vi "Diagnostics.Channel.Engine.vi"(8 "error in":errorcluster, 11 "State Variables":T1={"Comm"=refnum, "Parameters"={"Name"="", "CAN"={"Interface"="", "Baud Rate"=0, "Diagnostic Protocol"=enum."GMLAN", "Transport Protocol"=enum."ISO TP - Normal Mode", "Transmit ID"=0, "Receive ID"=2, "Transmit Extension"=1, "Receive Extension"=255, "Receive UUDT ID"=0, "Enable Stream"=TRUE, "VW TP Channel ID"=1, "Fill Frame"=FALSE, "Fill Byte"=0, "Termination"=FALSE, "LIN Cluster"="", "NAD"=8, "IO Mode"=0, "Max DLC"=0, "FD Baud Rate"=2, "Timeout"=1, "FD ISO Mode"=0, "DoIP Address"="", "DoIP Source Address"=3584, "DoIP Dynamic Port"=TRUE, "DoIP Version"=2}, "986x"={"Enable"=FALSE, "RIO Device"="", "Bitfile"=path ""}, "Reads"=[], "Frames Lookup"=variant(enum16{"GMLAN", "KWP-2000", "UDS"} enum."GMLAN"), "Writes"=[], "DPIDs"=[], "DPID Lookup"=variant(u32 0), "DTC"={"Descriptor"={"DTC Byte Length"=1, "Status Byte Length"=1, "Add Data Byte Length"=1, "Byte Order"=enum."Motorola"}, "Value.Code"=[], "Value.String"=[], "Value.J2012String"=[], "Status.Code"=[], "Status.String"=[]}, "Created DTCs"=0, "Polls"=[], "Service Channels Status Lookup"=variant, "Trigger Lookup"=variant, "Security"={"Type"=enum."None", "Source DLL Path"=path "", "Target DLL Path"=path "", "Security Level"=0, "Static Master Key"="", "Max Key Length"=1, "Host IP Address"=""}, "Initial Comm State"=FALSE}, "ADCS Connection"={"Diag CAN Handle"=0, "Transport Protocol"=enum."ISO TP - Normal Mode", "Receive Address Extension"=0, "Transmit Address Extension"=0, "Receive CAN Id"=0, "Transmit CAN Id"=0, "Log Frames ?"=FALSE, "My TP Address"=0, "Other TP Address"=0, "T1"=0, "T2"=0, "T3"=0, "T4"=0, "Tx SN"=0, "Block Size"=0, "Rx SN"=0, "VW TP Initialized?"=FALSE, "Tx block no"=0, "baud rate"=0, "Interface"="", "Channel Diag CAN Handle"=0, "UDP Connection ID"=refnum, "TCP Connection ID"=refnum, "Target IP Addr"=0, "Source Address"=0, "Target Address"=0, "Send Header NACK?"=FALSE, "DLL Handle"=0, "NAD"=0, "Time Stamp read first"=0.0, "Time Stamp read last"=0.0, "Time Stamp write first"=0.0, "Time Stamp write last"=0.0, "Time Stamp write"=0.0, "Time Stamp read"=0.0, " I/O Mode"=0, "FD Baudrate"=0, "TX_DL"=8, "RX_DL"=8, "DoIP Protocol Version"=1, " Selected I/O Mode"=0, "TesterPresent Counter"=0, "TesterPresent Limit"=0, "TesterPresent Tick[ms]"=10, "TesterPresent RequireResponse?"=FALSE, "TesterPresent Stored Ref?"=FALSE, "TesterPresent Message"=[], "TesterPresent Task Handle"=0, "TesterPresent Semaphore"=refnum, "Response Plausibility Check"=1, "Default Version?"=TRUE, "Diagostic Globals"={"Timeout FC (Bs)"=250, "Timeout CF (Cr)"=250, "Timeout Diag Command"=1000, "Receive Block Size (BS)"=0, "Wait Time CF (STmin)"=5, "Max Waits (N_WFTmax)"=10, "Waits to Send (N_WAIT)"=0, "Time between Waits (TW)"=25, "Fill CAN Frames?"=TRUE, "Fill Byte"=255, "Invalid Response as Error?"=FALSE, "Max RspPending Count"=5, "VWTP Command Timeout"=50, "Transport Protocol"=enum."Diagnostics on IP", "Diag CAN Handle"=0, "DLL Handle"=0, "Timeout RspPending"=1000}, "Session-based Properties?"=FALSE}, "XNET References"={"Database"="", "GMLAN.DPID.Frame"="", "Cluster.Convert"=""}, "XNETEngine (GMLAN)"=refnum, "Process"=refnum, "Reads"=refnum, "Writes"=refnum, "Cmds"=refnum, "DTCs"=refnum, "DTC Count"=refnum, "Status"=refnum, "Triggers"=refnum, "CANConnected"=refnum, "LocalStop"=refnum, "LocalCommStatus"=refnum, "Service Channels Status"=refnum, "Settings"=refnum, "Streaming Refs"={"Addon"="", "Port"="", "Filter Ref"=refnum, "Default Filter"={"ID Filters"=[], "Direction Filter"=enum."Tx/Rx", "Type Filter"=enum."All"}, "Port Settings"={"Mode"=0, "Baud Rate"=0, "Termination"=0, "FD ISO Mode"=0, "FD Baud Rate"=0}}} {"Streaming Refs"."Port Settings"."FD ISO Mode" items=["ISO", "Non ISO", "ISO Legacy"]; "Streaming Refs"."Port Settings"."Termination" items=["Off", "On"]; "Streaming Refs"."Port Settings"."Mode" items=["CAN 2.0", "CAN FD", "CAN FD+BRS"]; "ADCS Connection"."Diagostic Globals"."Fill Byte" format="%x"; "ADCS Connection"."TesterPresent Message" format="%.0x"; "ADCS Connection"."Selected I/O Mode" items=["CAN", "CAN FD", "CAN FD+BRS", "ECU Determined"]; "ADCS Connection"."DoIP Protocol Version" items=["2010"=1, "2012"=2]; "ADCS Connection"."RX_DL" items=["8"=8, "12"=12, "16"=16, "20"=20, "24"=24, "32"=32, "48"=48, "64"=64]; "ADCS Connection"."TX_DL" items=["8"=8, "12"=12, "16"=16, "20"=20, "24"=24, "32"=32, "48"=48, "64"=64]; "ADCS Connection"."I/O Mode" items=["CAN", "CAN FD", "CAN FD+BRS", "Not yet determined"]; "Parameters"."Writes"."Signals"."Byte Order" items=["Little Endian", "Big Endian"]; "Parameters"."Writes"."Signals"."Data Type" items=["Signed", "Unsigned", "IEEE Float"]; "Parameters"."CAN"."DoIP Version" items=["2010"=1, "2012"=2]; "Parameters"."CAN"."DoIP Source Address" format="%.0x"; "Parameters"."CAN"."FD ISO Mode" items=["ISO", "Non ISO", "ISO Legacy"]; "Parameters"."CAN"."IO Mode" items=["CAN 2.0", "CAN FD", "CAN FD+BRS"]; "Parameters"."CAN"."Fill Byte" format="%.0x"; "Parameters"."CAN"."VW TP Channel ID" format="%.0x"; "Parameters"."CAN"."Receive UUDT ID" format="%.0x"; "Parameters"."CAN"."Receive Extension" format="%.0x"; "Parameters"."CAN"."Transmit Extension" format="%.0x"; "Parameters"."CAN"."Receive ID" format="%.0x"; "Parameters"."CAN"."Transmit ID" format="%.0x"; "Parameters"."Reads"."Signals"."Byte Order" items=["Little Endian", "Big Endian"]; "Parameters"."Reads"."Signals"."Data Type" items=["Signed", "Unsigned", "IEEE Float"]}) -> (0 "error out":errorcluster)   [LabVIEW 2019, in "Diagnostics Addon Engine.lvlib"]
uses:
  Diagnostics Addon Engine.lvlib
  Types/Diagnostics.State.ctl
  <vilib>/NI/NIVS Inline Async API/_VS Inline Async API/Process/Process.lvclass
  <vilib>/NI/NI VeriStand Addon Network Comm/Engine/VeriStand Comm.lvclass
  Addon Shared/Types/SysDef.Compile.ctl
  Addon Shared/Types/CAN.ctl
  Addon Shared/Types/CAN.Interface.ctl
  Addon Shared/Types/Protocol.ctl
  Addon Shared/Types/Transport.ctl
  Addon Shared/Types/986x.ctl
  Addon Shared/Types/Frame.Compile.ctl
  Addon Shared/Types/Type.ctl
  Addon Shared/Types/Signal.ctl
  Addon Shared/Types/DPID.ctl
  Addon Shared/Types/DPID.Rate.ctl
  Addon Shared/Types/DTC.Settings.ctl
  Addon Shared/Types/DTC.Descriptor.ctl
  Addon Shared/Types/Poll.Compiled.ctl
  Addon Shared/Types/Security.ctl
  Addon Shared/Types/Security.Type.ctl
  <vilib>/Automotive Diagnostic Command Set/Diagnostic Transport.llb/Diag Reference.ctl
  <vilib>/Automotive Diagnostic Command Set/Diagnostic Transport.llb/Transport Protocol Selector.ctl
  <vilib>/Automotive Diagnostic Command Set/Diagnostic Transport.llb/DoIP Protocol Version.ctl
  <vilib>/Automotive Diagnostic Command Set/Diagnostic Transport.llb/Diag Globals.ctl
  Types/XNET.Refs.ctl
  <vilib>/NI/AMC/Message Queue.ctl
  <vilib>/NI/AMC/Message.ctl
  <vilib>/NI/Tools/Keyed Array/KeyedArray.ctl
  <vilib>/NI/NIVS Inline Async API/_Data Access Engine/Data Access Engine/Types/Write.DVR.ctl
  <vilib>/NI/NIVS Inline Async API/_Data Access Engine/Access Type Classes/Write/Write.lvclass
  <vilib>/NI/NIVS Inline Async API/_Data Access Engine/Data Access Engine/Types/Read.DVR.ctl
  <vilib>/NI/NIVS Inline Async API/_Data Access Engine/Access Type Classes/Read/Read.lvclass
  <vilib>/NI/NIVS Inline Async API/_Data Access Engine/Data Access Engine/Types/ReadWrite.DVR.ctl
  <vilib>/NI/NIVS Inline Async API/_Data Access Engine/Access Type Classes/ReadWrite/ReadWrite.lvclass
  SubModules/CAN-Streaming-Support/Source/Addon/Addon Engine/Types/Engine Stream Refs.ctl
  SubModules/CAN-Streaming-Support/Source/Addon/Addon Shared/Types/Direction Filter.ctl
  SubModules/CAN-Streaming-Support/Source/Addon/Addon Shared/Types/Type Filter.ctl
  SubModules/CAN-Streaming-Support/Source/Addon/Addon Shared/Types/Filter Parameters.ctl
  SubModules/CAN-Streaming-Support/Source/Addon/Addon Engine/Types/Engine Stream Port Settings.ctl
  <vilib>/NI/NIVS Inline Async API/_Data Access Engine/Access Type Classes/ReadWrite/ReadWrite.lvclass/ReadWrite.ctl
  Addon Shared/Types/Trigger.Settings.ctl
  <vilib>/NI/NI VeriStand Addon Network Comm/Engine/VeriStand Comm.lvclass/VeriStand Comm.ctl
  <vilib>/NI/NIVS Inline Async API/_Data Access Engine/Access Type Classes/Read/Read.lvclass/Read.ctl
  Types/Diagnostics.Command.ctl
  Addon Shared/Types/Command.New.ctl
  <vilib>/NI/NIVS Inline Async API/_VS Inline Async API/Process/Process.lvclass/Process.ctl
  <vilib>/NI/NIVS Inline Async API/_Data Access Engine/Data Access Engine/Methods/ReadWrite.Data.Read.vi
  <vilib>/NI/NIVS Inline Async API/_Data Access Engine/Data Access Engine/Methods/ReadWrite.Data.Reset.vi
  <vilib>/NI/NIVS Inline Async API/_Data Access Engine/Data Access Engine/Methods/Read.Data.vi
  <vilib>/NI/NIVS Inline Async API/_Data Access Engine/Access Type Classes/ReadWrite/ReadWrite.ProcessData.Read.vi
  <vilib>/NI/NIVS Inline Async API/_Data Access Engine/Access Type Classes/ReadWrite/ReadWrite.ProcessData.Reset.vi
  <vilib>/NI/AMC/Send Local Message.vi
  Addon Shared/SubVIs/Format ECU Master Key to String.vi
  <vilib>/NI/AMC/Send Local Messages.vi
  <vilib>/NI/NIVS Inline Async API/_Data Access Engine/Access Type Classes/Read/Read.ProcessData.vi
  <vilib>/NI/NIVS Inline Async API/_VS Inline Async API/Error Handling Process/SubVIs/Error.ConvertArray.vi
  <vilib>/NI/AMC/Create Single Message.vi
  <vilib>/NI/AMC/Update Message Routing Info.vi
  <vilib>/NI/AMC/Create Multiple Messages.vi
  <vilib>/NI/AMC/Send Message.vi
  <vilib>/NI/NIVS Inline Async API/_Data Access Engine/Data Access Engine/Data Access Engine.lvclass
  Addon Shared/Diagnostics Addon Shared.lvlib
  <vilib>/NI/Tools/Keyed Array/Tools_KeyedArray.lvlib
  <vilib>/NI/AMC/AMC.lvlib
  <vilib>/addons/Automotive Diagnostic Command Set/NI_Automotive Diagnostic Command Set.lvlib
  SubModules/CAN-Streaming-Support/Source/Addon/Addon Engine/CAN Stream Support Engine.lvlib
  SubModules/CAN-Streaming-Support/Source/Addon/Addon Shared/CAN Stream Support Shared.lvlib
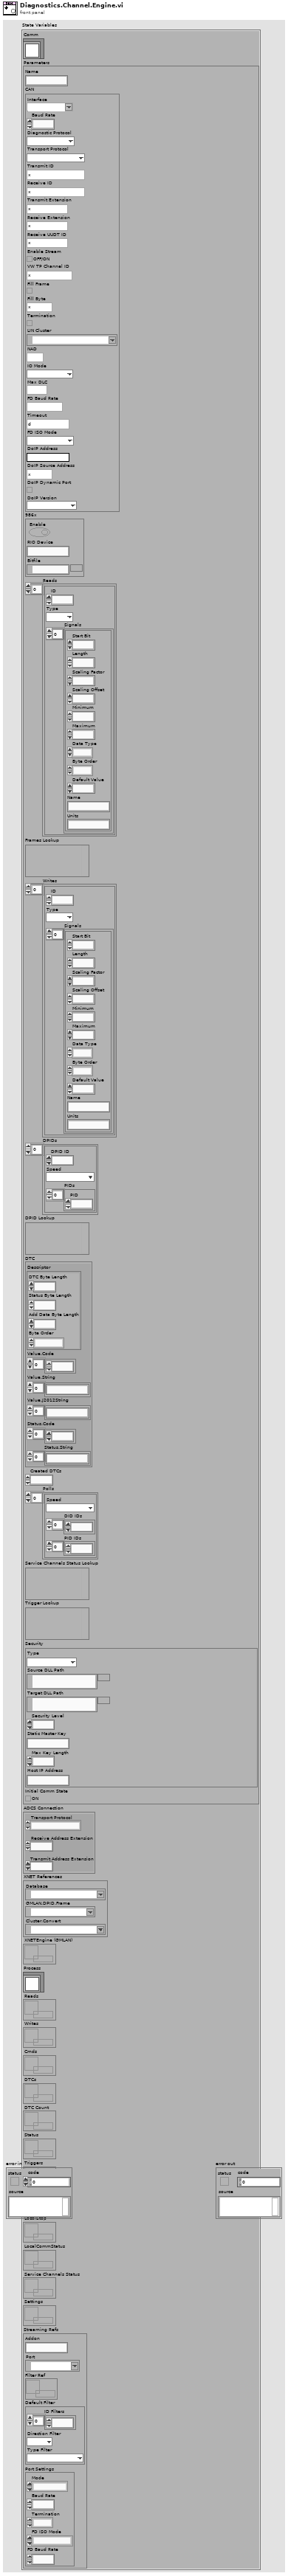
[diagram p1: front panel]
types:
  T1 = typedef "Diagnostics Addon Engine.lvlib/Diagnostics.State.ctl" = cluster{"Comm":refnum<class "VeriStand Comm.lvclass">, "Parameters":T2, "ADCS Connection":T18, "XNET References":T23, "XNETEngine (GMLAN)":T24, "Process":refnum<class "Process.lvclass">, "Reads":T25, "Writes":T26, "Cmds":T27, "DTCs":T25, "DTC Count":T25, "Status":T25, "Triggers":T27, "CANConnected":T25, "LocalStop":refnum<data-value>, "LocalCommStatus":refnum<data-value>, "Service Channels Status":T25, "Settings":T26, "Streaming Refs":T28}
  T2 = typedef "Diagnostics Addon Shared.lvlib/SysDef.Compile.ctl" = cluster{"Name":string, "CAN":T3, "986x":T7, "Reads":T8[], "Frames Lookup":variant, "Writes":T8[], "DPIDs":T11[], "DPID Lookup":variant, "DTC":T13, "Created DTCs":u32, "Polls":T15[], "Service Channels Status Lookup":variant, "Trigger Lookup":variant, "Security":T16, "Initial Comm State":bool}
  T3 = typedef "Diagnostics Addon Shared.lvlib/CAN.ctl" = cluster{"Interface":T4, "Baud Rate":u64, "Diagnostic Protocol":T5, "Transport Protocol":T6, "Transmit ID":u32, "Receive ID":u32, "Transmit Extension":u8, "Receive Extension":u8, "Receive UUDT ID":u32, "Enable Stream":bool, "VW TP Channel ID":u32, "Fill Frame":bool, "Fill Byte":u8, "Termination":bool, "LIN Cluster":refnum<k21>, "NAD":u8, "IO Mode":u32, "Max DLC":u16, "FD Baud Rate":u64, "Timeout":u32, "FD ISO Mode":u32, "DoIP Address":string, "DoIP Source Address":u16, "DoIP Dynamic Port":bool, "DoIP Version":u16}
  T4 = typedef "Diagnostics Addon Shared.lvlib/CAN.Interface.ctl" = string
  T5 = typedef "Diagnostics Addon Shared.lvlib/Protocol.ctl" = enum16{"GMLAN", "KWP-2000", "UDS", "User-Defined"}
  T6 = typedef "Diagnostics Addon Shared.lvlib/Transport.ctl" = enum16{"ISO TP - Normal Mode", "ISO TP - Mixed Mode", "VW TP 2.0", "Diagnostics on IP", "ISO TP LIN"}
  T7 = typedef "Diagnostics Addon Shared.lvlib/986x.ctl" = cluster{"Enable":bool, "RIO Device":string, "Bitfile":path}
  T8 = typedef "Diagnostics Addon Shared.lvlib/Frame.Compile.ctl" = cluster{"ID":u32, "Type":T9, "Signals":T10[]}
  T9 = typedef "Diagnostics Addon Shared.lvlib/Type.ctl" = enum16{"DID", "CDID", "PID", "CPID", "Read Memory", "Write Memory", "IO Control", "Routine Start", "Routine Request", "Routine Stop", "User Defined", "DTC Control", "Clear DTCs", "Read DTCs", "Start DTCs", "DTC Change Count", "Tester Present", "Unlock ECU", "Reset ECU", "Diag Session Control", "Communication Control", "DPID Control", "Poll Control", "Diag Comm Port Control"}
  T10 = typedef "Diagnostics Addon Shared.lvlib/Signal.ctl" = cluster{"Start Bit":u32, "Length":u32, "Scaling Factor":dbl, "Scaling Offset":dbl, "Minimum":dbl, "Maximum":dbl, "Data Type":u32, "Byte Order":u32, "Default Value":dbl, "Name":string, "Units":string}
  T11 = typedef "Diagnostics Addon Shared.lvlib/DPID.ctl" = cluster{"DPID ID":u8, "Speed":T12, "PIDs":u16[]}
  T12 = typedef "Diagnostics Addon Shared.lvlib/DPID.Rate.ctl" = enum16{"Slow", "Medium", "Fast"}
  T13 = typedef "Diagnostics Addon Shared.lvlib/DTC.Settings.ctl" = cluster{"Descriptor":T14, "Value.Code":dbl[], "Value.String":string[], "Value.J2012String":string[], "Status.Code":dbl[], "Status.String":string[]}
  T14 = typedef "Diagnostics Addon Shared.lvlib/DTC.Descriptor.ctl" = cluster{"DTC Byte Length":i32, "Status Byte Length":i32, "Add Data Byte Length":i32, "Byte Order":enum16{"Motorola", "Intel"}}
  T15 = typedef "Diagnostics Addon Shared.lvlib/Poll.Compiled.ctl" = cluster{"Speed":T12, "DID IDs":u32[], "PID IDs":u32[]}
  T16 = typedef "Diagnostics Addon Shared.lvlib/Security.ctl" = cluster{"Type":T17, "Source DLL Path":path, "Target DLL Path":path, "Security Level":u8, "Static Master Key":string, "Max Key Length":u32, "Host IP Address":string}
  T17 = typedef "Diagnostics Addon Shared.lvlib/Security.Type.ctl" = enum16{"None", "SeedKey DLL", "MasterKey (Channel)", "MasterKey (Static)", "SeedKey DLL (Windows)"}
  T18 = typedef "NI_Automotive Diagnostic Command Set.lvlib/Diag Reference.ctl" = cluster{"Diag CAN Handle":u32, "Transport Protocol":T19, "Receive Address Extension":u8, "Transmit Address Extension":u8, "Receive CAN Id":u32, "Transmit CAN Id":u32, "Log Frames ?":bool, "My TP Address":u8, "Other TP Address":u8, "T1":u16, "T2":u16, "T3":u16, "T4":u16, "Tx SN":u8, "Block Size":u8, "Rx SN":u8, "VW TP Initialized?":bool, "Tx block no":u8, "baud rate":u64, "Interface":string, "Channel Diag CAN Handle":u32, "UDP Connection ID":refnum<k16>, "TCP Connection ID":refnum<k5>, "Target IP Addr":u32, "Source Address":u16, "Target Address":u16, "Send Header NACK?":bool, "DLL Handle":u32, "NAD":u8, "Time Stamp read first":dbl, "Time Stamp read last":dbl, "Time Stamp write first":dbl, "Time Stamp write last":dbl, "Time Stamp write":dbl, "Time Stamp read":dbl, " I/O Mode":u32, "FD Baudrate":u64, "TX_DL":u16, "RX_DL":u16, "DoIP Protocol Version":T20, " Selected I/O Mode":u32, "TesterPresent Counter":u32, "TesterPresent Limit":u32, "TesterPresent Tick[ms]":i32, "TesterPresent RequireResponse?":bool, "TesterPresent Stored Ref?":bool, "TesterPresent Message":u8[], "TesterPresent Task Handle":i32, "TesterPresent Semaphore":T21, "Response Plausibility Check":u32, "Default Version?":bool, "Diagostic Globals":T22, "Session-based Properties?":bool}
  T19 = typedef "NI_Automotive Diagnostic Command Set.lvlib/Transport Protocol Selector.ctl" = enum16{"ISO TP - Normal Mode", "ISO TP - Mixed Mode", "VW TP 2.0", "Diagnostics on IP", "ISO TP LIN"}
  T20 = typedef "NI_Automotive Diagnostic Command Set.lvlib/DoIP Protocol Version.ctl" = u8
  T21 = typedef "Semaphore RefNum" = refnum<k1>
  T22 = typedef "NI_Automotive Diagnostic Command Set.lvlib/Diag Globals.ctl" = cluster{"Timeout FC (Bs)":u32, "Timeout CF (Cr)":u32, "Timeout Diag Command":u32, "Receive Block Size (BS)":u8, "Wait Time CF (STmin)":u8, "Max Waits (N_WFTmax)":u8, "Waits to Send (N_WAIT)":i32, "Time between Waits (TW)":u32, "Fill CAN Frames?":bool, "Fill Byte":u32, "Invalid Response as Error?":bool, "Max RspPending Count":u32, "VWTP Command Timeout":u32, "Transport Protocol":T19, "Diag CAN Handle":u32, "DLL Handle":u32, "Timeout RspPending":u32}
  T23 = typedef "Diagnostics Addon Engine.lvlib/XNET.Refs.ctl" = cluster{"Database":refnum<k21>, "GMLAN.DPID.Frame":refnum<k21>, "Cluster.Convert":refnum<k21>}
  T24 = typedef "AMC.lvlib/Message Queue.ctl" = refnum<queue>
  T25 = typedef "Data Access Engine.lvlib/Data Access Engine.lvclass/Write.DVR.ctl" = refnum<data-value>
  T26 = typedef "Data Access Engine.lvlib/Data Access Engine.lvclass/Read.DVR.ctl" = refnum<data-value>
  T27 = typedef "Data Access Engine.lvlib/Data Access Engine.lvclass/ReadWrite.DVR.ctl" = refnum<data-value>
  T28 = typedef "CAN Stream Support Engine.lvlib/Engine Stream Refs.ctl" = cluster{"Addon":string, "Port":refnum<k21>, "Filter Ref":refnum<data-value>, "Default Filter":T29, "Port Settings":T32}
  T29 = typedef "CAN Stream Support Shared.lvlib/Filter Parameters.ctl" = cluster{"ID Filters":u32[], "Direction Filter":T30, "Type Filter":T31}
  T30 = typedef "CAN Stream Support Shared.lvlib/Direction Filter.ctl" = enum16{"Tx/Rx", "Rx", "Tx"}
  T31 = typedef "CAN Stream Support Shared.lvlib/Type Filter.ctl" = enum16{"All", "CAN Data", "CAN Remote", "CAN Bus Error", "CAN 2.0 Data", "CAN FD Data", "CAN FD+BRS Data", "J1939 Data", "Delay", "Log Trigger", "Start Trigger"}
  T32 = typedef "CAN Stream Support Engine.lvlib/Engine Stream Port Settings.ctl" = cluster{"Mode":u32, "Baud Rate":u64, "Termination":u32, "FD ISO Mode":u32, "FD Baud Rate":u64}
  T33 = typedef "Diagnostics Addon Shared.lvlib/Trigger.Settings.ctl" = cluster{"Type":T9, "ID":u32, "Settings?":bool, "Index":i32, "Length":i32}
  T34 = typedef "Diagnostics Addon Engine.lvlib/Diagnostics.Command.ctl" = enum8{"None", "Clear Status Channels", "Read DIDs", "Read DID", "Write DID", "Read PIDs", "Read PID", "Write CPID", "Write Memory", "Read Memory", "Input Output Control", "Start Routine", "Request Routine Status", "Stop Routine", "Configure and Start DPIDs", "Stop DPIDs", "Start DTCs", "Read DTCs", "Clear DTCs", "Control DTC", "Read Failure Record Parameters", "Enable Change DTC Count", "Disable Change DTC Count", "Restart Communication", "Close Communication", "Force Tester Present", "Enable Repeating Tester Present", "Disable Repeating Tester Present", "Unlock ECU", "ECU Reset", "Enable Diagnostic Session", "Disable Diagnostic Session", "Disable Normal Communication", "Return To Normal Mode", "Pass Thru Channel Based", "Start Polling", "Stop Polling"}
  T35 = typedef "Diagnostics Addon Shared.lvlib/Command.New.ctl" = enum8{"None", "Clear Status Channels", "Read All DIDs", "Read All PIDs", "Configure and Start DPIDs", "Stop DPIDs"}
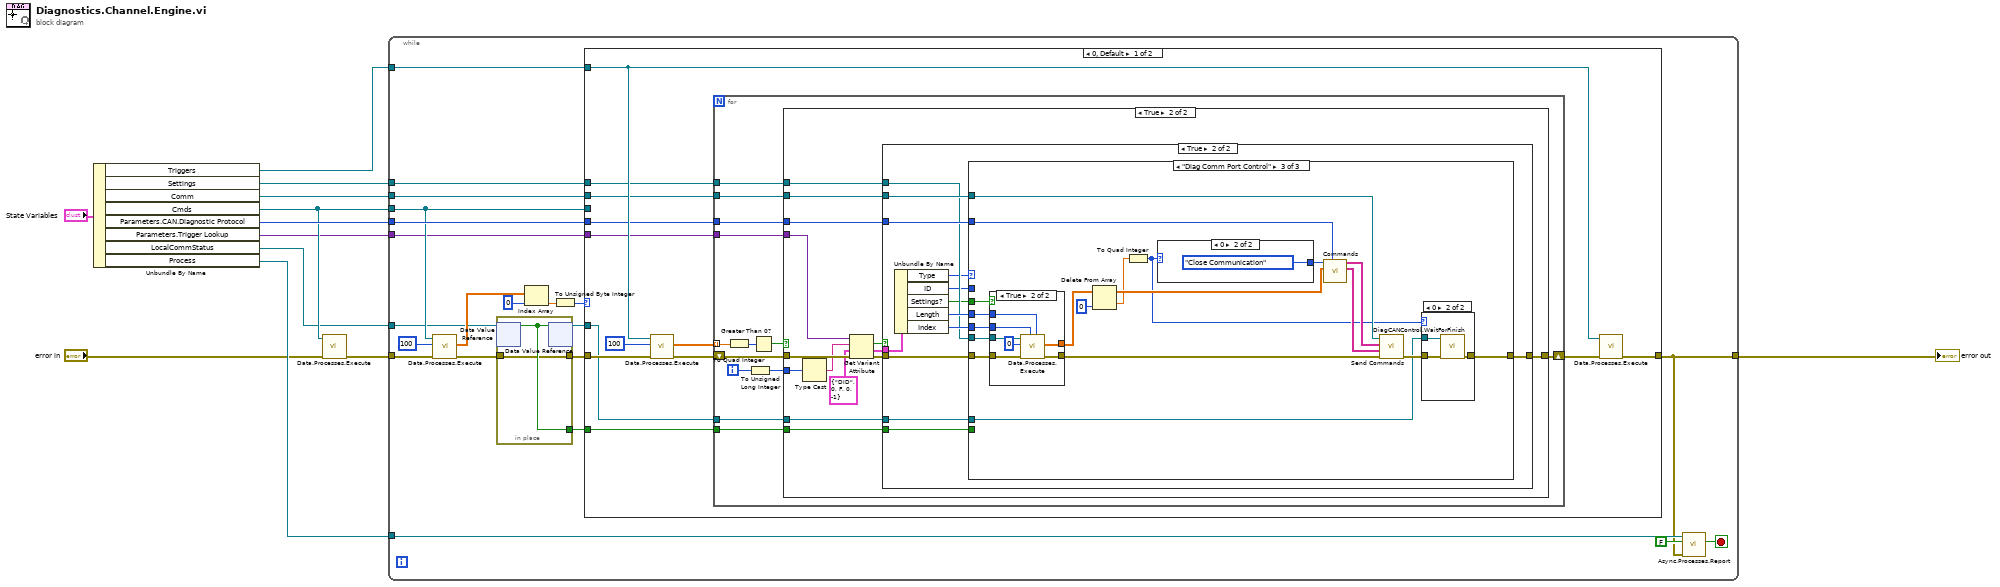
[diagram p0: block diagram]
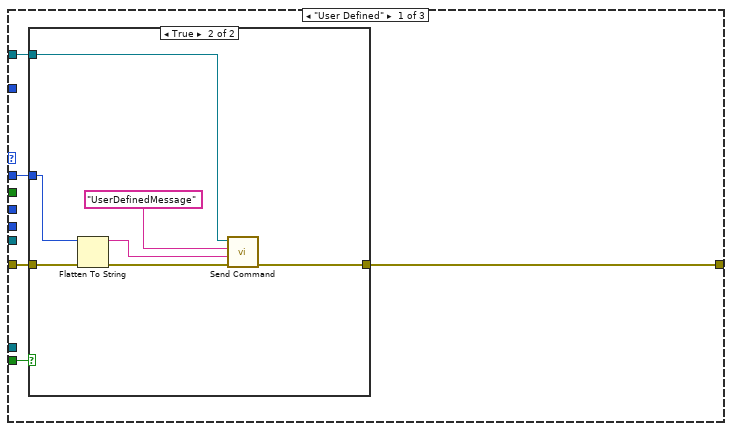
[diagram p4: hidden frame]
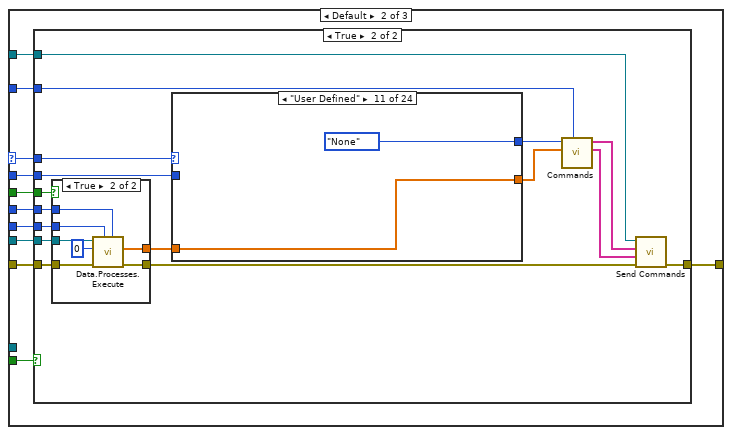
[diagram p6: hidden frame]
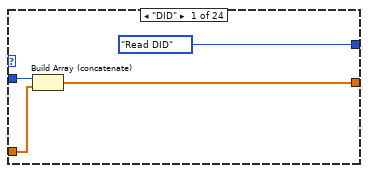
[diagram p8: hidden frame]
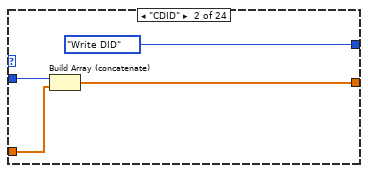
[diagram p9: hidden frame]
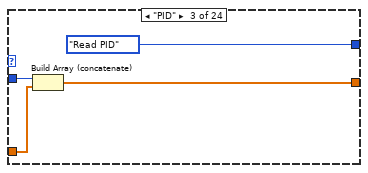
[diagram p10: hidden frame]
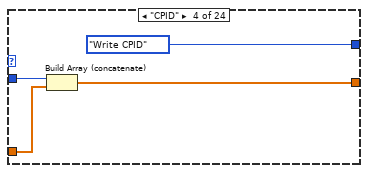
[diagram p11: hidden frame]
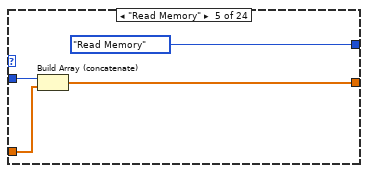
[diagram p12: hidden frame]
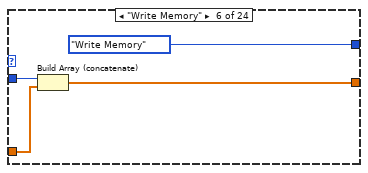
[diagram p13: hidden frame]
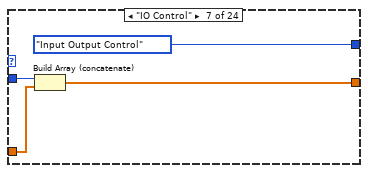
[diagram p14: hidden frame]
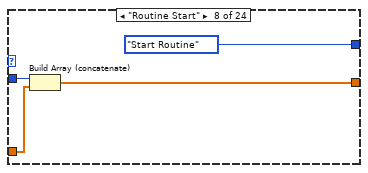
[diagram p15: hidden frame]
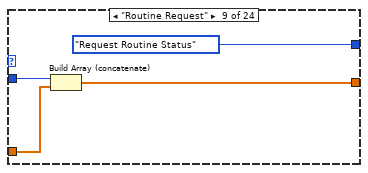
[diagram p16: hidden frame]
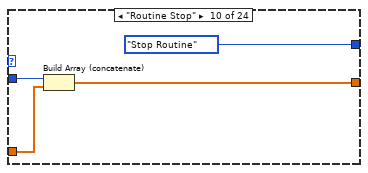
[diagram p17: hidden frame]
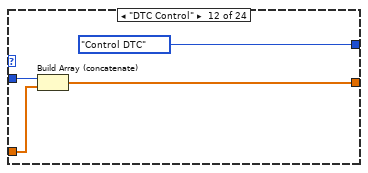
[diagram p18: hidden frame]
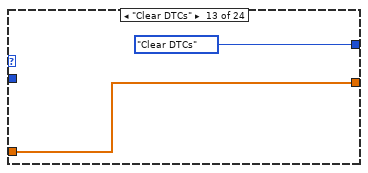
[diagram p19: hidden frame]
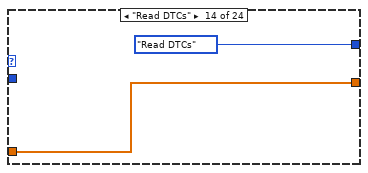
[diagram p20: hidden frame]
diagram:
  n1 = Unbundle By Name("State Variables") -> ("Triggers"=w7:T27, "Settings"=w2:T26, "Comm"=w9:refnum<class "VeriStand Comm.lvclass">, "Cmds"=w4:T27, "Parameters.CAN.Diagnostic Protocol"=w8:T5, "Parameters.Trigger Lookup"=w1:variant, "LocalCommStatus"=w3:refnum<data-value>, "Process"=w11:refnum<class "Process.lvclass">)
  n2 = call-poly <vilib>:"Data.Processes.Execute.vi"("error in (no error)"="error in", "Ref"=w4) -> ("error out"=w5:errorcluster)  [unwired: 8 in, 1 out]
  n3 = while {
    tunnel: w4 -> [w25]
    tunnel: w11 -> [w30]
    tunnel: [w24] -> w10
    tunnel: w5 -> [w26]
    tunnel: w9 -> [w33]
    tunnel: w8 -> [w32]
    tunnel: w7 -> [w29]
    tunnel: w3 -> [w19]
    tunnel: w2 -> [w17]
    tunnel: w1 -> [w16]
    stop <- w23 stop-if-true
    n4 = call-poly <vilib>:"Data.Processes.Execute.vi"("error in (no error)"=w26, "timeout ms"=100 ("timeout in ms (0)"), "Ref"=w25) -> ("error out"=w21:errorcluster, "Data"=w27:dbl[])  [unwired: 5 in, 2 out]
    n5 = in-place {
      in-place-border: [w35] -> w20
      in-place-border: [w34] -> w22
      in-place-border: w21 -> [w34]
      n6 = in-place-dvr #1(w19) -> (w35:bool)  [unwired: 1 out]
      n7 = in-place-dvr #1(w35) -> (w18:refnum<data-value>)  [unwired: 1 out]
    }
    n8 = Index Array(array=w27, index=0) -> (element=w14:dbl)
    n9 = To Unsigned Byte Integer(number=w14) -> (unsigned 8bit integer=w13:u8)
    n10 = case shown="0, Default" w13 {
      selector: w13 -> [_ w294]
      tunnel: w22 -> [w43 w297]
      tunnel: [w41 w292] -> w24
      tunnel: w33 -> [w42 w296]
      tunnel: w32 -> [w40 w295]
      tunnel: w29 -> [w44 _]
      tunnel: w25 -> [_ w289]
      tunnel: w20 -> [w36 w291]
      tunnel: w18 -> [w37 _]
      tunnel: w17 -> [w39 _]
      tunnel: w16 -> [w38 _]
      frame 0, Default {
        n11 = call-poly <vilib>:"Data.Processes.Execute.vi"("error in (no error)"=w43, "timeout ms"=100 ("timeout in ms (0)"), "Ref"=w44) -> ("error out"=w47:errorcluster, "Data"=w46:dbl[])  [unwired: 5 in, 2 out]
        n12 = for {
          shift-right: [w57] -> w45
          shift-left: w47 -> [w58]
          tunnel: w46 -> [w61] mode=indexing
          tunnel: w40 -> [w56]
          tunnel: w42 -> [w55]
          tunnel: w39 -> [w54]
          tunnel: w38 -> [w53]
          tunnel: w37 -> [w51]
          tunnel: w36 -> [w50]
          i -> [w52]
          n13 = To Quad Integer(1:w61) -> (0:w60:i64)
          n14 = To Unsigned Long Integer(number=w52) -> (unsigned 32bit integer=w49:u32)
          n15 = Greater Than 0?(x=w60) -> (x > 0?=w59:bool)
          n16 = case shown="True" w59 {
            tunnel: w58 -> [w62 w76]
            tunnel: [w62 w69] -> w57
            tunnel: w49 -> [_ w75]
            tunnel: w56 -> [_ w70]
            tunnel: w55 -> [_ w68]
            tunnel: w54 -> [_ w67]
            tunnel: w53 -> [_ w66]
            tunnel: w51 -> [_ w64]
            tunnel: w50 -> [_ w63]
            frame False {
            }
            frame True {
              n17 = Type Cast(x=w75) -> (*(type *) &x=w74:string)  [unwired: 1 in]
              n18 = Get Variant Attribute(Variant=w66, name=w74, default value (empty Variant)=T33 {"Type"=enum."DID", "ID"=0, "Settings?"=FALSE, "Index"=0, "Length"=-1}, error in=w76) -> (found=w65:bool, value=w72:T33, error out=w71:errorcluster)  [unwired: 1 out]
              n19 = case shown="True" w65 {
                tunnel: w72 -> [_ w90]
                tunnel: w71 -> [w77 w87]
                tunnel: w70 -> [_ w86]
                tunnel: [w77 w85] -> w69
                tunnel: w68 -> [_ w84]
                tunnel: w67 -> [_ w83]
                tunnel: w64 -> [_ w79]
                tunnel: w63 -> [_ w78]
                frame False {
                }
                frame True {
                  n20 = Unbundle By Name(w90) -> ("Type"=w81:T9, "ID"=w80:u32, "Settings?"=w82:bool, "Length"=w88:i32, "Index"=w89:i32)
                  n21 = case shown="\"Diag Comm Port Control\"" w81 {
                    selector: w81 -> [_ w106 _]
                    tunnel: w89 -> [_ w114 w274]
                    tunnel: w88 -> [_ w113 w273]
                    tunnel: w87 -> [w92 w112 w272]
                    tunnel: w86 -> [_ w111 w270]
                    tunnel: [w95 w110 w258] -> w85
                    tunnel: w84 -> [w94 w109 w267]
                    tunnel: w83 -> [_ w108 w266]
                    tunnel: w82 -> [_ w107 w265]
                    tunnel: w80 -> [w93 w105 _]
                    tunnel: w79 -> [_ _ w257]
                    tunnel: w78 -> [w91 w104 _]
                    frame "User Defined" {
                      n22 = case shown="True" w91 {
                        tunnel: [w96 w103] -> w95
                        tunnel: w94 -> [_ w102]
                        tunnel: w93 -> [_ w100]
                        tunnel: w92 -> [w96 w98]
                        frame False {
                        }
                        frame True {
                          n23 = Flatten To String(anything=w100, error in (no error)=w98) -> (data string=w97:string, error out=w99:errorcluster)  [unwired: 2 in, 1 out]
                          n24 = call <vilib>:"Send Command.vi"("error in (no error)"=w99, "message value"=w97, "message name"="UserDefinedMessage", "VeriStand Comm in"=w102) -> ("error out"=w103:errorcluster)  [unwired: 6 in, 1 out]
                        }
                      }
                    }
                    frame Default {
                      n25 = case shown="True" w104 {
                        tunnel: w114 -> [_ w131]
                        tunnel: w113 -> [_ w130]
                        tunnel: w112 -> [w115 w129]
                        tunnel: w111 -> [_ w127]
                        tunnel: [w115 w126] -> w110
                        tunnel: w109 -> [_ w123]
                        tunnel: w108 -> [_ w122]
                        tunnel: w107 -> [_ w121]
                        tunnel: w106 -> [_ w120]
                        tunnel: w105 -> [_ w117]
                        frame False {
                        }
                        frame True {
                          n26 = case shown="True" w121 {
                            tunnel: w131 -> [_ w255]
                            tunnel: w130 -> [_ w254]
                            tunnel: w129 -> [w248 w253]
                            tunnel: [_ w251] -> w118
                            tunnel: [w248 w250] -> w128
                            tunnel: w122 -> [_ w249]
                            frame False {
                            }
                            frame True {
                              n27 = call-poly <vilib>:"Data.Processes.Execute.vi"("length"=w254, "index"=w255, "error in (no error)"=w253, "timeout ms"=0, "Ref"=w249) -> ("error out"=w250:errorcluster, "Values"=w251:dbl[])  [unwired: 4 in, 1 out]
                            }
                          }
                          n28 = case shown="\"User Defined\"" w120 {
                            tunnel: [Diagnostics.Command."Read DID" ("Enum") Diagnostics.Command."Write DID" ("Enum") Diagnostics.Command."Read PID" ("Enum") Diagnostics.Command."Write CPID" ("Enum") Diagnostics.Command."Read Memory" ("Enum") Diagnostics.Command."Write Memory" ("Enum") Diagnostics.Command."Input Output Control" ("Enum") Diagnostics.Command."Start Routine" ("Enum") Diagnostics.Command."Request Routine Status" ("Enum") Diagnostics.Command."Stop Routine" ("Enum") Diagnostics.Command."None" ("Enum") Diagnostics.Command."Control DTC" ("Enum") Diagnostics.Command."Clear DTCs" ("Enum") Diagnostics.Command."Read DTCs" ("Enum") Diagnostics.Command."Start DTCs" ("Enum") w189 w192 Diagnostics.Command."Unlock ECU" ("Enum") Diagnostics.Command."ECU Reset" ("Enum") w204 w212 w223 w233 w240] -> w119
                            tunnel: w118 -> [w133 w137 w141 w145 w149 w153 w157 w161 w165 w169 w172 w175 w178 w180 w182 w188 w194 w200 w202 w206 w214 w224 w234 w242]
                            tunnel: w117 -> [w134 w138 w142 w146 w150 w154 w158 w162 w166 w170 _ w176 _ _ _ _ _ _ _ _ _ w222 w232 _]
                            tunnel: [w132 w136 w140 w144 w148 w152 w156 w160 w164 w168 w172 w174 w178 w180 w182 w186 w193 w200 w202 w205 w213 w220 w230 w241] -> w116
                            frame "DID" {
                              n29 = Build Array (concatenate)(w134, w133) -> (w132:dbl[])
                            }
                            frame "CDID" {
                              n30 = Build Array (concatenate)(w138, w137) -> (w136:dbl[])
                            }
                            frame "PID" {
                              n31 = Build Array (concatenate)(w142, w141) -> (w140:dbl[])
                            }
                            frame "CPID" {
                              n32 = Build Array (concatenate)(w146, w145) -> (w144:dbl[])
                            }
                            frame "Read Memory" {
                              n33 = Build Array (concatenate)(w150, w149) -> (w148:dbl[])
                            }
                            frame "Write Memory" {
                              n34 = Build Array (concatenate)(w154, w153) -> (w152:dbl[])
                            }
                            frame "IO Control" {
                              n35 = Build Array (concatenate)(w158, w157) -> (w156:dbl[])
                            }
                            frame "Routine Start" {
                              n36 = Build Array (concatenate)(w162, w161) -> (w160:dbl[])
                            }
                            frame "Routine Request" {
                              n37 = Build Array (concatenate)(w166, w165) -> (w164:dbl[])
                            }
                            frame "Routine Stop" {
                              n38 = Build Array (concatenate)(w170, w169) -> (w168:dbl[])
                            }
                            frame "User Defined" {
                            }
                            frame "DTC Control" {
                              n39 = Build Array (concatenate)(w176, w175) -> (w174:dbl[])
                            }
                            frame "Clear DTCs" {
                            }
                            frame "Read DTCs" {
                            }
                            frame "Start DTCs" {
                            }
                            frame "DTC Change Count" {
                              n40 = Delete From Array(array=w188, index=0) -> (deleted portion=w185:dbl, array with subset deleted=w186:dbl[])  [unwired: 1 in]
                              n41 = To Quad Integer(1:w185) -> (0:w184:i64)
                              n42 = case shown="0" w184 {
                                tunnel: [Diagnostics.Command."Enable Change DTC Count" ("Enum") Diagnostics.Command."Disable Change DTC Count" ("Enum")] -> w189
                                frame Default {
                                }
                                frame 0 {
                                }
                              }
                            }
                            frame "Tester Present" {
                              n43 = Delete From Array(array=w194, index=0) -> (deleted portion=w196:dbl, array with subset deleted=w193:dbl[])  [unwired: 1 in]
                              n44 = To Quad Integer(1:w196) -> (0:w195:i64)
                              n45 = case shown="0" w195 {
                                tunnel: [Diagnostics.Command."Enable Repeating Tester Present" ("Enum") Diagnostics.Command."Disable Repeating Tester Present" ("Enum")] -> w192
                                frame Default {
                                }
                                frame 0 {
                                }
                              }
                            }
                            frame "Unlock ECU" {
                            }
                            frame "Reset ECU" {
                            }
                            frame "Diag Session Control" {
                              n46 = Delete From Array(array=w206, index=0) -> (deleted portion=w208:dbl, array with subset deleted=w205:dbl[])  [unwired: 1 in]
                              n47 = To Quad Integer(1:w208) -> (0:w207:i64)
                              n48 = case shown="Default" w207 {
                                tunnel: [Diagnostics.Command."Enable Diagnostic Session" ("Enum") Diagnostics.Command."Disable Diagnostic Session" ("Enum")] -> w204
                                frame Default {
                                }
                                frame 0 {
                                }
                              }
                            }
                            frame "Communication Control" {
                              n49 = Delete From Array(array=w214, index=0) -> (deleted portion=w216:dbl, array with subset deleted=w213:dbl[])  [unwired: 1 in]
                              n50 = To Quad Integer(1:w216) -> (0:w215:i64)
                              n51 = case shown="0" w215 {
                                tunnel: [Diagnostics.Command."Return To Normal Mode" ("Enum") Diagnostics.Command."Disable Normal Communication" ("Enum")] -> w212
                                frame Default {
                                }
                                frame 0 {
                                }
                              }
                            }
                            frame "Poll Control" {
                              n52 = Delete From Array(array=w224, index=0) -> (deleted portion=w226:dbl, array with subset deleted=w221:dbl[])  [unwired: 1 in]
                              n53 = To Quad Integer(1:w226) -> (0:w225:i64)
                              n54 = case shown="0" w225 {
                                tunnel: [Diagnostics.Command."Start Polling" ("Enum") Diagnostics.Command."Stop Polling" ("Enum")] -> w223
                                frame Default {
                                }
                                frame 0 {
                                }
                              }
                              n55 = Build Array (concatenate)(w222, w221) -> (w220:dbl[])
                            }
                            frame "DPID Control" {
                              n56 = Delete From Array(array=w234, index=0) -> (deleted portion=w236:dbl, array with subset deleted=w231:dbl[])  [unwired: 1 in]
                              n57 = To Quad Integer(1:w236) -> (0:w235:i64)
                              n58 = case shown="Default" w235 {
                                tunnel: [Diagnostics.Command."Configure and Start DPIDs" ("Enum") Diagnostics.Command."Stop DPIDs" ("Enum")] -> w233
                                frame Default {
                                }
                                frame 0 {
                                }
                              }
                              n59 = Build Array (concatenate)(w232, w231) -> (w230:dbl[])
                            }
                            frame "Diag Comm Port Control" {
                              n60 = Delete From Array(array=w242, index=0) -> (deleted portion=w244:dbl, array with subset deleted=w241:dbl[])  [unwired: 1 in]
                              n61 = To Quad Integer(1:w244) -> (0:w243:i64)
                              n62 = case shown="0" w243 {
                                tunnel: [Diagnostics.Command."Restart Communication" ("Enum") Diagnostics.Command."Close Communication" ("Enum")] -> w240
                                frame Default {
                                }
                                frame 0 {
                                }
                              }
                            }
                          }
                          n63 = call "Commands.vi"("Diagnostic Protocol"=w127, "Data"=w116, "Enum"=w119) -> ("MetaData"=w125:string[], "Commands"=w124:string[])  [unwired: 7 in]
                          n64 = call <vilib>:"Send Commands.vi"("error in (no error)"=w128, "message values"=w125, "message names"=w124, "VeriStand Comm in"=w123) -> ("error out"=w126:errorcluster)  [unwired: 6 in, 1 out]
                        }
                      }
                    }
                    frame "Diag Comm Port Control" {
                      n65 = case shown="True" w265 {
                        tunnel: w274 -> [_ w288]
                        tunnel: w273 -> [_ w287]
                        tunnel: w272 -> [w281 w286]
                        tunnel: [_ w284] -> w263
                        tunnel: [w281 w283] -> w271
                        tunnel: w266 -> [_ w282]
                        frame False {
                        }
                        frame True {
                          n66 = call-poly <vilib>:"Data.Processes.Execute.vi"("length"=w287, "index"=w288, "error in (no error)"=w286, "timeout ms"=0, "Ref"=w282) -> ("error out"=w283:errorcluster, "Values"=w284:dbl[])  [unwired: 4 in, 1 out]
                        }
                      }
                      n67 = Delete From Array(array=w263, index=0) -> (deleted portion=w260:dbl, array with subset deleted=w262:dbl[])  [unwired: 1 in]
                      n68 = To Quad Integer(1:w260) -> (0:w256:i64)
                      n69 = case shown="0" w256 {
                        tunnel: [Diagnostics.Command."Restart Communication" ("Enum") Diagnostics.Command."Close Communication" ("Enum")] -> w264
                        frame Default {
                        }
                        frame 0 {
                        }
                      }
                      n70 = call "Commands.vi"("Diagnostic Protocol"=w270, "Data"=w262, "Enum"=w264) -> ("MetaData"=w269:string[], "Commands"=w268:string[])  [unwired: 7 in]
                      n71 = call <vilib>:"Send Commands.vi"("error in (no error)"=w271, "message values"=w269, "message names"=w268, "VeriStand Comm in"=w267) -> ("error out"=w259:errorcluster)  [unwired: 6 in, 1 out]
                      n72 = case shown="0" w256 {
                        tunnel: w259 -> [w275 w278]
                        tunnel: [w275 w277] -> w258
                        tunnel: w257 -> [_ w276]
                        frame Default {
                        }
                        frame 0 {
                          n73 = call "DiagCANControl.WaitForFinish.vi"("error in (no error)"=w278, "Data Value Reference in"=w276) -> ("error out"=w277:errorcluster)  [unwired: 9 in]
                        }
                      }
                    }
                  }
                }
              }
            }
          }
        }
        n74 = call-poly <vilib>:"Data.Processes.Execute.vi"("error in (no error)"=w45, "Ref"=w44) -> ("error out"=w41:errorcluster)  [unwired: 8 in, 1 out]
      }
      frame 1..5 {
        n75 = case shown="True" w291 {
          tunnel: w297 -> [w298 w310]
          tunnel: w296 -> [_ w307]
          tunnel: w295 -> [_ w304]
          tunnel: w294 -> [_ w303]
          tunnel: [w298 w306] -> w293
          tunnel: [w299 w305] -> w290
          tunnel: w289 -> [w299 w305]
          frame False {
          }
          frame True {
            n76 = Type Cast(type=Command.New."Stop DPIDs", x=w303) -> (*(type *) &x=w301:T35)
            n77 = case shown="\"Read All DIDs\"" w301 {
              tunnel: [Diagnostics.Command."None" Diagnostics.Command."Clear Status Channels" Diagnostics.Command."Read DIDs" Diagnostics.Command."Read PIDs" Diagnostics.Command."Configure and Start DPIDs" Diagnostics.Command."Stop DPIDs"] -> w300
              frame "None" {
              }
              frame "Clear Status Channels" {
              }
              frame "Read All DIDs" {
              }
              frame "Read All PIDs" {
              }
              frame "Configure and Start DPIDs" {
              }
              frame "Stop DPIDs" {
              }
            }
            n78 = call "Commands.vi"("Diagnostic Protocol"=w304, "Enum"=w300) -> ("MetaData"=w308:string[], "Commands"=w309:string[])  [unwired: 8 in]
            n79 = call <vilib>:"Send Commands.vi"("error in (no error)"=w310, "message values"=w308, "message names"=w309, "VeriStand Comm in"=w307) -> ("error out"=w306:errorcluster)  [unwired: 6 in, 1 out]
          }
        }
        n80 = call-poly <vilib>:"Data.Processes.Execute.vi"("error in (no error)"=w293, "Ref"=w290) -> ("error out"=w292:errorcluster)  [unwired: 8 in, 1 out]
      }
    }
    n81 = call <vilib>:"Async.Processes.Report.vi"("Error"=w24, "Stop Async on Error?"=FALSE ("Stop on Error?"), "Process in"=w30) -> ("Stop"=w23:bool)  [unwired: 7 in, 1 out]
  }
  "error out" <- w10
